vi "WriteImageDataToMap.vi"(4 "image timestamp":timestamp, 6 "image status":bool, 7 "map":T1, 8 "error in (no error)":errorcluster, 9 "image height":i32, 10 "image width":i32, 11 "image data":sgl[](array[numeric])) -> (0 "error out":errorcluster, 5 "map out":T1)   [LabVIEW 2017]
uses:
  <vilib>/addons/PointValueMap/controls/PointMap.ctl
  <vilib>/addons/PointValueMap/subVIs/Point_Write_variant.vi
  <vilib>/addons/PointValueMap/subVIs/Point_Write_i32.vi
  <vilib>/addons/PointValueMap/subVIs/Point_Write_string.vi
  <vilib>/addons/PointValueMap/PointValueMap.lvlib
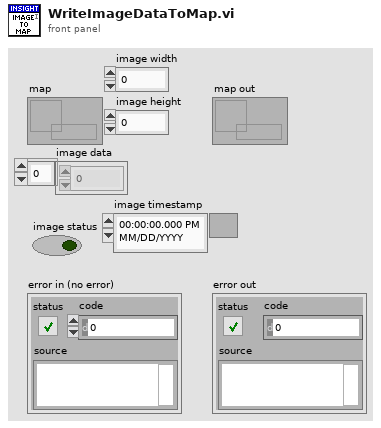
[diagram p1: front panel]
types:
  T1 = typedef "PointValueMap.lvlib/PointMap.ctl" = refnum<data-value>
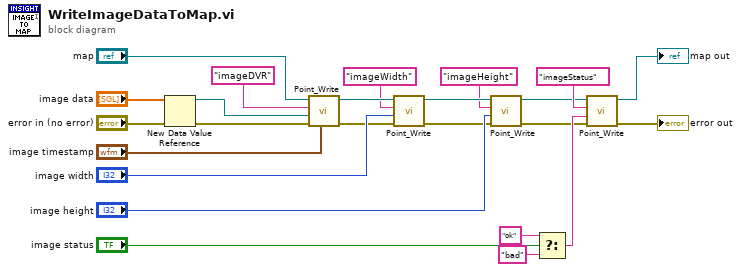
[diagram p0: block diagram]
diagram:
  n1 = New Data Value Reference(data value="image data", error in="error in (no error)") -> (data value reference=w12:refnum<data-value>, error out=w14:errorcluster)
  n2 = call-poly <vilib>:"Point_Write.vi"("Time Stamp"="image timestamp", "Error In"=w14, "Value"=w12, "Tag"="imageDVR", "Map"="map") -> ("Error Out"=w4:errorcluster, "Map Out"=w11:T1)  [unwired: 5 in]
  n3 = call-poly <vilib>:"Point_Write.vi"("Error In"=w4, "Value"="image width", "Tag"="imageWidth", "Map"=w11) -> ("Error Out"=w3:errorcluster, "Map Out"=w10:T1)  [unwired: 6 in]
  n4 = call-poly <vilib>:"Point_Write.vi"("Error In"=w3, "Value"="image height", "Tag"="imageHeight", "Map"=w10) -> ("Error Out"=w2:errorcluster, "Map Out"=w9:T1)  [unwired: 6 in]
  n5 = Select(t="ok", s="image status", f="bad") -> (s? t:f=w17:string)
  n6 = call-poly <vilib>:"Point_Write.vi"("Error In"=w2, "Value"=w17, "Tag"="imageStatus", "Map"=w9) -> ("Error Out"=→"error out":errorcluster, "Map Out"=→"map out":T1)  [unwired: 6 in]
